vi "Format command.vi"(8 "error in (no error)":errorcluster, 11 "Cluster":T1={"Command"=enum."£ncal", "data"=variant}) -> (0 "error out":errorcluster, 3 "String":string)   [LabVIEW 2016]
uses:
  Controls/Command cluster.ctl
  Controls/Command list.ctl
panel:
  out "No tokens":i32
  in  "input string":string
  out "Token String":string[](array[string])
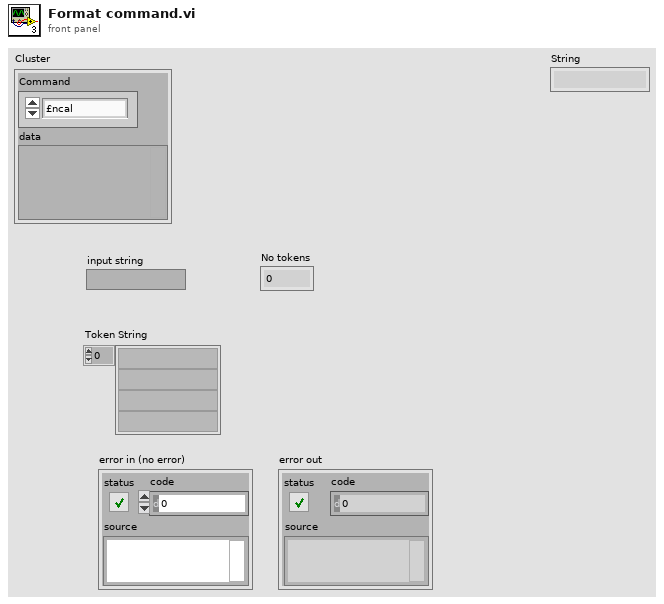
[diagram p1: front panel]
types:
  T1 = typedef "Command cluster.ctl" = cluster{"Command":T2, "data":variant}
  T2 = typedef "Command list.ctl" = enum16{"", "£nabort", "getaxisno", "£getserialno", "£nidentify", "&&£setnlimit", "&£nm", "&£snv", "&£speed", "£np", "£ncal"}
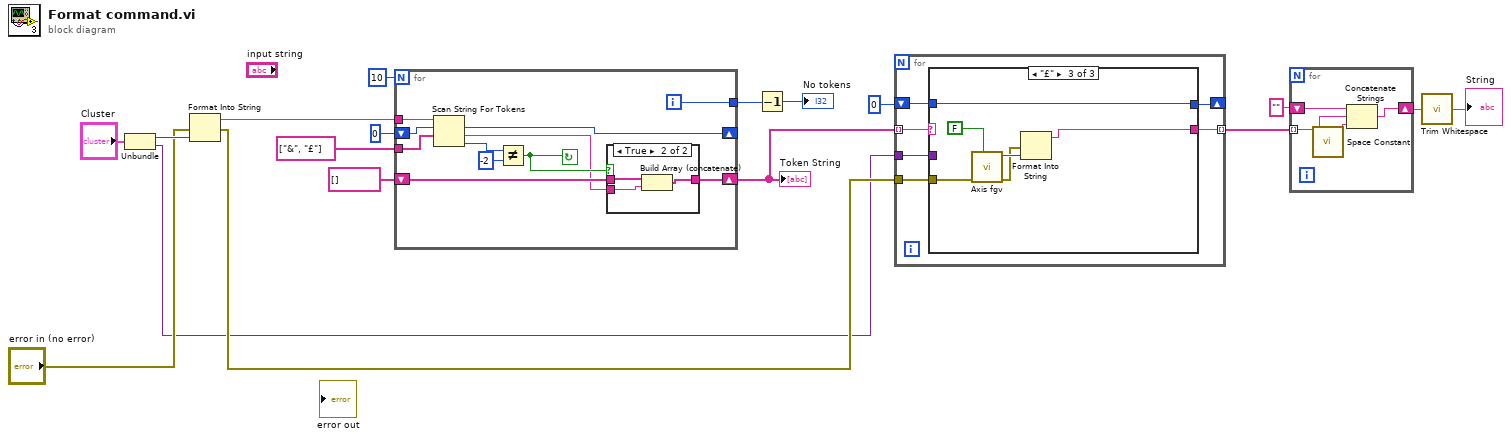
[diagram p0: block diagram]
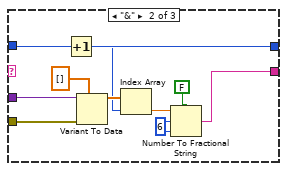
[diagram p3: hidden frame]
diagram:
  n1 = Unbundle("Cluster") -> ("Command"=w5:T2, "data"=w1:variant)
  n2 = Format Into String(error in="error in (no error)", w5) -> (resulting string=w4:string, error out=w2:errorcluster)  [unwired: 2 in]
  n3 = for {
    N: 10 -> [_]
    shift-right: [w27] -> _
    shift-left: 0 ("offset past token") -> [w29]
    tunnel: string[] ["&", "£"] ("delimiters (\\s,\\t,\\r,\\n)") -> [w25]
    shift-right: [w21] -> w12
    shift-left: string[] [] -> [w23]
    tunnel: w4 -> [w20]
    tunnel: [w19] -> w14
    i -> [w19]
    stop <- w24 continue-if-true
    n4 = Scan String For Tokens(7:w25, 8:w29, 9:w20) -> (0:w28:i32, 1:w22:string, 2:w27:i32)  [unwired: 3 in, 1 out]
    n5 = Not Equal?(x=w28, y=-2) -> (x != y?=w24:bool)
    n6 = case shown="True" w24 {
      tunnel: w23 -> [w30 w33]
      tunnel: w22 -> [_ w32]
      tunnel: [w30 w31] -> w21
      frame False {
      }
      frame True {
        n7 = Build Array (concatenate)(w33, w32) -> (w31:string[])
      }
    }
  }
  "Token String" <- w12
  n8 = Decrement(x=w14) -> (x-1=→"No tokens":i32)
  n9 = for {
    tunnel: w12 -> [w39] mode=indexing
    tunnel: w1 -> [w38]
    shift-right: [w36] -> _
    shift-left: 0 -> [w37]
    tunnel: w2 -> [w35]
    tunnel: [w34] -> w10 mode=indexing
    n10 = case shown="\"£\"" w39 {
      selector: w39 -> [w41 _ _]
      tunnel: w38 -> [_ w48 _]
      tunnel: w37 -> [w40 w44 w57]
      tunnel: [w40 w49 w57] -> w36
      tunnel: w35 -> [_ w47 w56]
      tunnel: [w41 w42 w53] -> w34
      frame "False", Default {
      }
      frame "&" {
        w50 = i16 6 ("width (-)")
        n11 = Increment(x=w44) -> (x+1=w49:i32)
        n12 = Variant To Data(error in=w47, type=dbl[] [], Variant=w48) -> (data=w45:dbl[])  [unwired: 1 out]
        n13 = Index Array(array=w45, index=w44) -> (element=w43:dbl)
        n14 = Number To Fractional String(use system decimal point (T)=FALSE, number=w43, width (-)=w50, precision (6)=w50) -> (F-format string=w42:string)
      }
      frame "£" {
        n15 = call "Axis fgv.vi"("Set"=FALSE, "error in (no error)"=w56) -> ("error out"=w54:errorcluster, "Axis out"=w55:u16)  [unwired: 8 in]
        n16 = Format Into String(error in=w54, w55) -> (resulting string=w53:string)  [unwired: 2 in, 1 out]
      }
    }
  }
  n17 = for {
    tunnel: w10 -> [w60] mode=indexing
    shift-right: [w58] -> w8
    shift-left: "" -> [w61]
    n18 = call <vilib>:"Space Constant.vi"() -> ("String"=w59:string)
    n19 = Concatenate Strings(w61, w60, w59) -> (w58:string)
  }
  n20 = call <vilib>:"Trim Whitespace.vi"("string"=w8) -> ("trimmed string"=→"String":string)  [unwired: 1 in]
